vi "Initialize FEMC.vi"(9 "Slave Node in":cluster{"Address":i16, "Serial Number":i8[]} {"Serial Number" format="%.0x"; "Address" format="%.0x"}, 10 "Cartridge band":u32=1 min=1 max=10 step=1, 11 "ObjHandle in":u32) -> (0 "error out":errorcluster caption="エラー出力", 2 "Info String":string)   [LabVIEW 2017]
panel:
  # "ALMA Monitor and Control Bus\nInitialize FEMC"
  # "にエラー出力追加\n2009.9.11　藤井"
  # "Node Address"
  # "Serial Number"
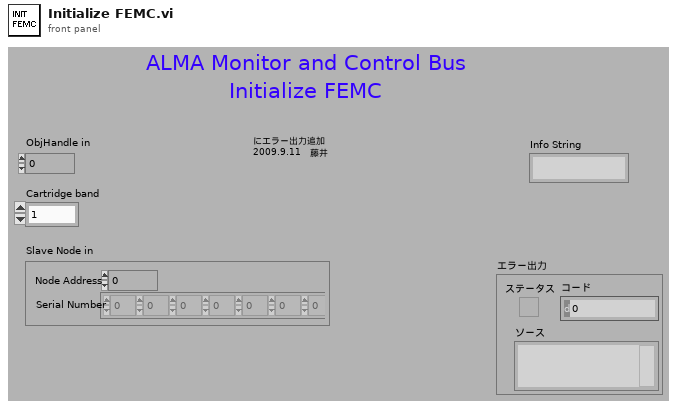
[diagram p1: front panel]
types:
  T1 = cluster{"Data Array out[0]":u8, "Data Array out[1]":u8, "Data Array out[2]":u8, "Data Array out[3]":u8, "Data Array out[4]":u8, "Data Array out[5]":u8, "Data Array out[6]":u8, "Data Array out[7]":u8}
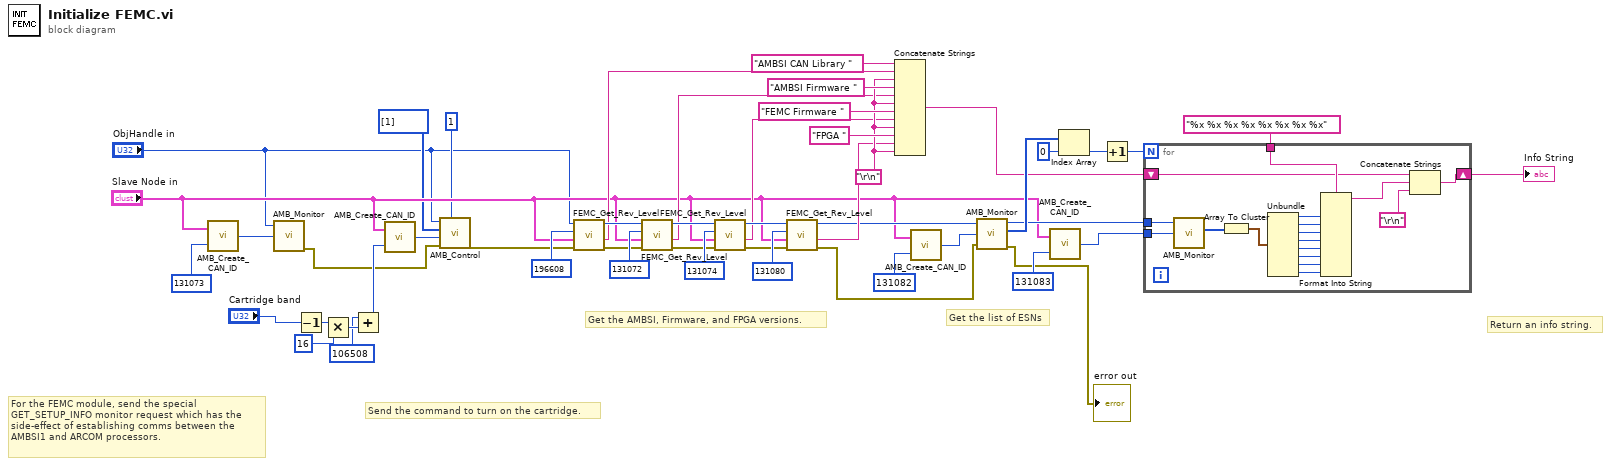
[diagram p0: block diagram]
diagram:
  w33 = "\r\n"
  # "Send the command to turn on the cartridge."
  # "Return an info string."
  # "Get the list of ESNs"
  # "Get the AMBSI, Firmware, and FPGA versions."
  # "For the FEMC module, send the special\nGET_SETUP_INFO monitor request which has the\nside-effect of establishing comms between the \nAMBSI1 and ARCOM processors."
  n1 = call "AMB_Create_CAN_ID.vi"("Relative Address in"=u32 131073, "Slave Node in"="Slave Node in") -> ("CAN ID out"=w48:u32)
  n2 = call "AMB_Monitor.vi"("ObjHandle in"="ObjHandle in", "CAN ID in"=w48) -> ("error out"=w3:errorcluster)  [unwired: 1 in, 3 out]
  n3 = Decrement(x="Cartridge band") -> (x-1=w13:u32)
  n4 = Multiply(x=w13, y=16) -> (x*y=w11:u32)
  n5 = Add(x=u32 106508 ("Relative Address in"), y=w11) -> (x+y=w10:u32)
  n6 = call "AMB_Create_CAN_ID.vi"("Relative Address in"=w10, "Slave Node in"="Slave Node in") -> ("CAN ID out"=w9:u32)
  n7 = call "AMB_Control.vi"("ObjHandle in"="ObjHandle in", "Data in"=u8[] [1], "CAN ID in"=w9, "error in"=w3, "Data Length in"=u8 1) -> ("error out"=w4:errorcluster)  [unwired: 1 out]
  n8 = call "FEMC_Get_Rev_Level.vi"("error in"=w4, "Slave Node in"="Slave Node in", "RCA"=u32 196608 ("Relative Address in"), "ObjHandle in"="ObjHandle in") -> ("error out"=w40:errorcluster, "Revision Level out"=w29:string, "ObjHandle out"=w47:u32)  [unwired: 1 in]
  n9 = call "FEMC_Get_Rev_Level.vi"("error in"=w40, "Slave Node in"="Slave Node in", "RCA"=u32 131072 ("Relative Address in"), "ObjHandle in"=w47) -> ("error out"=w39:errorcluster, "Revision Level out"=w30:string, "ObjHandle out"=w46:u32)  [unwired: 1 in]
  n10 = call "FEMC_Get_Rev_Level.vi"("error in"=w39, "Slave Node in"="Slave Node in", "RCA"=u32 131074 ("Relative Address in"), "ObjHandle in"=w46) -> ("error out"=w38:errorcluster, "Revision Level out"=w31:string, "ObjHandle out"=w45:u32)  [unwired: 1 in]
  n11 = call "FEMC_Get_Rev_Level.vi"("error in"=w38, "Slave Node in"="Slave Node in", "RCA"=u32 131080 ("Relative Address in"), "ObjHandle in"=w45) -> ("error out"=w2:errorcluster, "Revision Level out"=w32:string, "ObjHandle out"=w26:u32)  [unwired: 1 in]
  n12 = Concatenate Strings("AMBSI CAN Library " ("string"), w29, w33, "AMBSI Firmware " ("string"), w30, w33, "FEMC Firmware " ("string"), w31, w33, "FPGA " ("string"), w32, w33) -> (w19:string)
  n13 = call "AMB_Create_CAN_ID.vi"("Relative Address in"=u32 131082, "Slave Node in"="Slave Node in") -> ("CAN ID out"=w27:u32)
  n14 = call "AMB_Monitor.vi"("ObjHandle in"=w26, "CAN ID in"=w27, "error in"=w2) -> ("ObjHandle out"=w21:u32, "Data Array out"=w24:u8[], "error out"=→"error out":errorcluster)  [unwired: 1 out]
  n15 = call "AMB_Create_CAN_ID.vi"("Relative Address in"=u32 131083, "Slave Node in"="Slave Node in") -> ("CAN ID out"=w22:u32)
  n16 = Index Array(array=w24, index=0) -> (element=w15:u8)
  n17 = Increment(x=w15) -> (x+1=w14:u8)
  n18 = for {
    N: w14 -> [_]
    tunnel: w22 -> [w66]
    tunnel: w21 -> [w65]
    tunnel: "%x %x %x %x %x %x %x %x" ("format string") -> [w54]
    shift-right: [w50] -> w18
    shift-left: w19 -> [w51]
    n19 = call "AMB_Monitor.vi"("ObjHandle in"=w65, "CAN ID in"=w66) -> ("Data Array out"=w64:u8[])  [unwired: 1 in, 3 out]
    n20 = Array To Cluster(array=w64) -> (cluster=w63:T1)
    n21 = Unbundle(w63) -> ("Data Array out[0]"=w62:u8, "Data Array out[1]"=w61:u8, "Data Array out[2]"=w60:u8, "Data Array out[3]"=w59:u8, "Data Array out[4]"=w58:u8, "Data Array out[5]"=w57:u8, "Data Array out[6]"=w56:u8, "Data Array out[7]"=w55:u8)
    n22 = Format Into String(format string=w54, w62, w61, w60, w59, w58, w57, w56, w55) -> (resulting string=w52:string)  [unwired: 2 in, 1 out]
    n23 = Concatenate Strings(w51, w52, "\r\n") -> (w50:string)
  }
  "Info String" <- w18
